vi "Example.vi"   [LabVIEW 2014]
uses:
  TableLogger_Actor/TableLoggerConfig.ctl
  TableLogger_Actor/TableLoggerTypes.ctl
  TableLogger_Actor/Messages/InsertData_Msg/InsertData_Msg.lvclass/InsertData_Msg.ctl
  <vilib>/ActorFramework/Message Enqueuer/Message Enqueuer.lvclass/Message Enqueuer.ctl
  <vilib>/ActorFramework/Message Enqueuer/Enqueue.vi
  <vilib>/ActorFramework/Message Priority Queue/Priority Enqueue.vi
  TableLogger_Actor/Messages/InsertData_Msg/InsertData_Msg.lvclass
  <vilib>/ActorFramework/Stop Msg/Stop Msg.lvclass
  TableLogger_Actor/TableLogger_Actor/TableLogger_Actor.lvclass
  TableLogger_Actor/TableLogger_Actor.lvlib
panel:
  # "Look at the block diagram for details about this VI"
types:
  T1 = cluster{"Numeric Data":i32, "Float Data":dbl, "String Data":string, "Enum Data":enum16{"Enum Item 1", "Enum Item 2"}, "Array Data":i32[]}
  T2 = typedef "TableLogger_Actor.lvlib/TableLoggerConfig.ctl" = cluster{"TableLogger":T3, "DB File Path":path, "DB Backup Interval (Hours)":i32, "Max DB Size (MB)":i32, "Backup Directory":path}
  T3 = typedef "TableLogger_Actor.lvlib/TableLoggerTypes.ctl" = enum16{"CSV Logger", "SQLite Logger"}
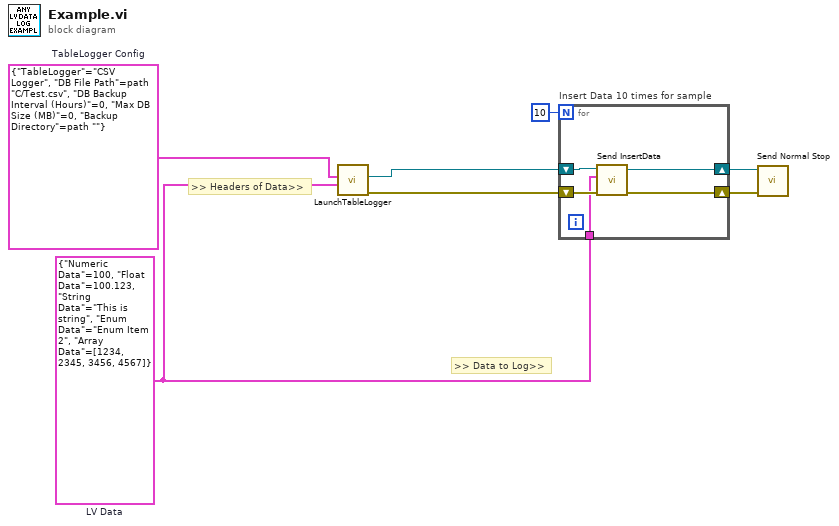
[diagram p0: block diagram]
diagram:
  w1 = T1 {"Numeric Data"=100, "Float Data"=100.123, "String Data"="This is string", "Enum Data"=enum."Enum Item 2", "Array Data"=[1234, 2345, 3456, 4567]}  # LV Data
  w6 = T2 {"TableLogger"=enum."CSV Logger", "DB File Path"=path "C:/Test.csv", "DB Backup Interval (Hours)"=0, "Max DB Size (MB)"=0, "Backup Directory"=path ""}  # TableLogger Config
  # ">> Headers of Data>>"
  # ">> Data to Log>>"
  n1 = call "LaunchTableLogger.vi"("Data Cluster (for Headers)"=w1, "TableLogger Config"=w6) -> ("error out"=w5:errorcluster, "TableLogger Actor's Enqueuer"=w7:refnum<class "Message Enqueuer.lvclass">)  [unwired: 6 in, 2 out]
  n2 = for "Insert Data 10 times for sample" {
    N: 10 -> [_]
    shift-right: [w9] -> w3
    shift-left: w7 -> [w12]
    shift-right: [w10] -> w4
    shift-left: w5 -> [w11]
    tunnel: w1 -> [w8]
    n3 = call "Send InsertData.vi"("error in (no error)"=w11, "Data"=w8, "Message Enqueuer"=w12) -> ("error out"=w10:errorcluster, "Message Enqueuer out"=w9:refnum<class "Message Enqueuer.lvclass">)  [unwired: 7 in]
  }
  n4 = call <vilib>:"Send Normal Stop.vi"("error in (no error)"=w4, "Message Enqueuer"=w3) -> ()  [unwired: 9 in, 1 out]
